vi "h5_save_image.vi"(4 "array":i16[][](array[numeric]), 7 "TYPE":string="IMG", 9 "Attributes":T1, 10 "SQUID":string="100", 11 "H5":path[](array[path])=[path ""]) -> (0 "error out":errorcluster)   [LabVIEW 2015, in "camera.lvlib"]
uses:
  <vilib>/UPVI/lvhdf5/dataset.llb/LVH5D Operation.ctl
  <vilib>/UPVI/lvhdf5/dataset.llb/Simple OpenCreateReplace Dataset (Variant).vi
  <vilib>/Utility/VariantDataType/GetClusterInfo.vi
  <vilib>/Utility/VariantDataType/GetTypeInfo.vi
  <vilib>/UPVI/lvhdf5/attribute.llb/Write Multiple Attributes.vi
  <vilib>/UPVI/lvhdf5/dataset.llb/Append Element(s) to Dataset (Variant).vi
  <vilib>/UPVI/lvhdf5/dataset.llb/Simple OpenCreateReplace Dataset.xnode
  <vilib>/UPVI/lvhdf5/library.llb/HDF5 Ref.ctl
  <vilib>/UPVI/lvhdf5/attribute.llb/LVH5A Operation.ctl
  <vilib>/UPVI/lvhdf5/attribute.llb/LVH5 Write Attributes.xnode
  <vilib>/UPVI/lvhdf5/attribute.llb/Cluster to Attribute Array.xnode
  <vilib>/UPVI/lvhdf5/dataset.llb/Append Element(s) to Dataset.xnode
  camera.lvlib
  oskar_tools/oskar_tools.lvlib
  <vilib>/Utility/VariantDataType/VariantType.lvlib
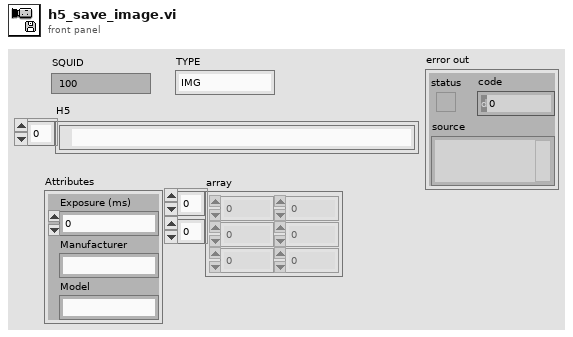
[diagram p1: front panel]
types:
  T1 = cluster{"Exposure (ms)":i32, "Manufacturer":string, "Model":string}
  T2 = typedef "Semaphore RefNum" = refnum<k1>
  T3 = typedef "LVH5D Operation.ctl" = enum16{"open", "replace", "create", "open or create", "create or replace", "create or replace with confirmation"}
  T4 = typedef "HDF5 Ref.ctl" = refnum<k1>
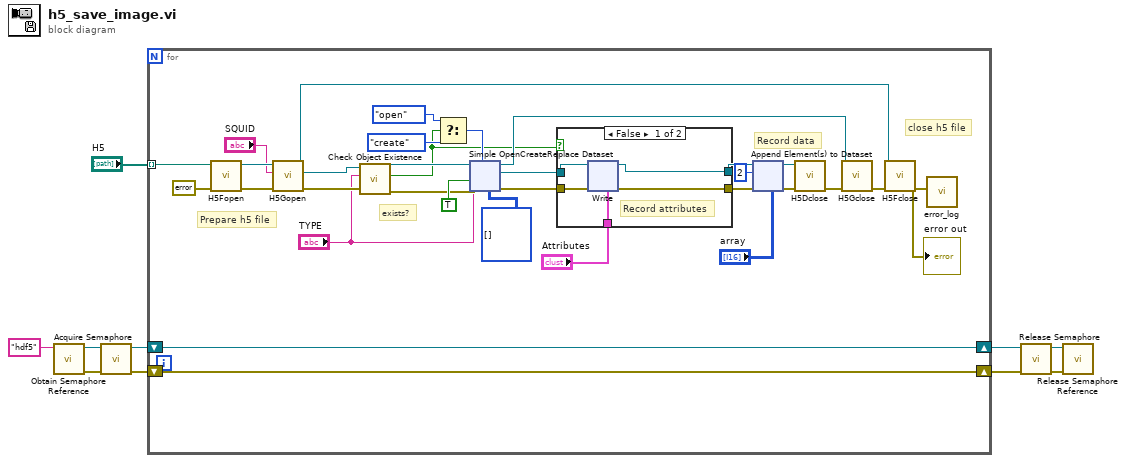
[diagram p0: block diagram]
diagram:
  n1 = call <vilib>:"Obtain Semaphore Reference.vi"("name (unnamed)"="hdf5") -> ("error out"=w8:errorcluster, "semaphore"=w9:T2)  [unwired: 4 in, 1 out]
  n2 = call <vilib>:"Acquire Semaphore.vi"("error in (no error)"=w8, "semaphore"=w9) -> ("error out"=w3:errorcluster, "semaphore out"=w4:T2)  [unwired: 3 in, 1 out]
  n3 = for {
    tunnel: "H5" -> [w40] mode=indexing
    shift-right: [w41] -> w2
    shift-left: w4 -> [w41]
    shift-right: [w42] -> w1
    shift-left: w3 -> [w42]
    # "exists?"
    # "Record data"
    # "close h5 file"
    # "Prepare h5 file"
    n4 = call <vilib>:"H5Fopen.vi"("error in (no error)"=errorcluster {"status"=FALSE, "code"=0, "source"=""} ("error out"), "path"=w40) -> ("error out"=w38:errorcluster, "HDF5 Ref out"=w37:T4)  [unwired: 6 in]
    n5 = call <vilib>:"H5Gopen.vi"("error in (no error)"=w38, "Name"="SQUID", "HDF5 Ref"=w37) -> ("error out"=w32:errorcluster, "HDF5 Group Ref"=w33:T4, "HDF5 Ref out"=w35:T4)  [unwired: 4 in]
    n6 = call <vilib>:"Check Object Existence.vi"("error in (no error)"=w32, "name"="TYPE", "HDF5 Ref"=w33) -> ("error out"=w25:errorcluster, "Exists"=w17:bool, "HDF5 Ref out"=w24:T4)  [unwired: 4 in]
    n7 = Select(t=LVH5D_Operation."open" ("operation"), s=w17, f=LVH5D_Operation."create" ("operation")) -> (s? t:f=w21:T3)
    n8 = xnode "Simple OpenCreateReplace Dataset"("Dataset Path"="TYPE", "HDF5 Ref"=w24, "Unlimited  dataset (F)"=TRUE, "error in (no error)"=w25, "operation"=w21, "Datatype and Dataspace"=i16[][][] [] ("array 2")) -> ("HDF5 Dataset Ref out"=w16:T4, "HDF5 Ref out"=w30:T4, "error out"=w20:errorcluster)  [unwired: 2 in]
    n9 = case shown="False" w17 {
      tunnel: w20 -> [w47 w167]
      tunnel: [w45 w167] -> w19
      tunnel: [w44 w166] -> w18
      tunnel: w16 -> [w46 w166]
      tunnel: "Attributes" -> [w43 _]
      frame False {
        # "Record attributes"
        n10 = xnode "Write"("HDF5 Ref"=w46, "error in (no error)"=w47, "Value(s)"=w43) -> ("HDF5 Ref out"=w44:T4, "error out"=w45:errorcluster)  [unwired: 2 in]
      }
      frame True {
      }
    }
    n11 = xnode "Append Element(s) to Dataset"("Dimension to Extend (0)"=2, "HDF5 Dataset Ref"=w18, "error in (no error)"=w19, "Data Element(s)"="array") -> ("HDF5 Dataset out"=w26:T4, "error out"=w27:errorcluster)  [unwired: 2 out]
    n12 = call <vilib>:"H5Dclose.vi"("error in (no error)"=w27, "HDF5 Dataset Ref"=w26) -> ("error out"=w31:errorcluster)  [unwired: 7 in]
    n13 = call <vilib>:"H5Gclose.vi"("error in (no error)"=w31, "HDF5 Group Ref"=w30) -> ("error out"=w36:errorcluster)  [unwired: 7 in]
    n14 = call <vilib>:"H5Fclose.vi"("error in (no error)"=w36, "HDF5 Ref"=w35) -> ("error out"=w34:errorcluster)  [unwired: 7 in]
    "error out" <- w34
    n15 = call "error_log.vi"("error"=w34) -> ()  [unwired: 10 in]
  }
  n16 = call <vilib>:"Release Semaphore.vi"("error in (no error)"=w1, "semaphore"=w2) -> ("error out"=w6:errorcluster, "semaphore out"=w5:T2)  [unwired: 4 in]
  n17 = call <vilib>:"Release Semaphore Reference.vi"("error in (no error)"=w6, "semaphore"=w5) -> ()  [unwired: 8 in, 2 out]
